vi "HW_Detect_compatible_COM_ports.vi"(0 "Retrieval method (NI-VISA)":enum16{"NI-VISA", "WMIC"}(ring), 1 "Error In":errorcluster) -> (2 "Detected COM ports":T1[](array[typedef]), 3 "Output string from CMD":string="\r\r\n\r\r\n", 4 "Standard error output from CMD":string="No Instance(s) Available.\r\r\n", 5 "Error Out":errorcluster)   [LabVIEW 2018, in "Common_Resources.lvlib"]
uses:
  SubVi's/Controls/CTL_VISA_port_Descr.-Name.ctl
  Common_Resources.lvlib
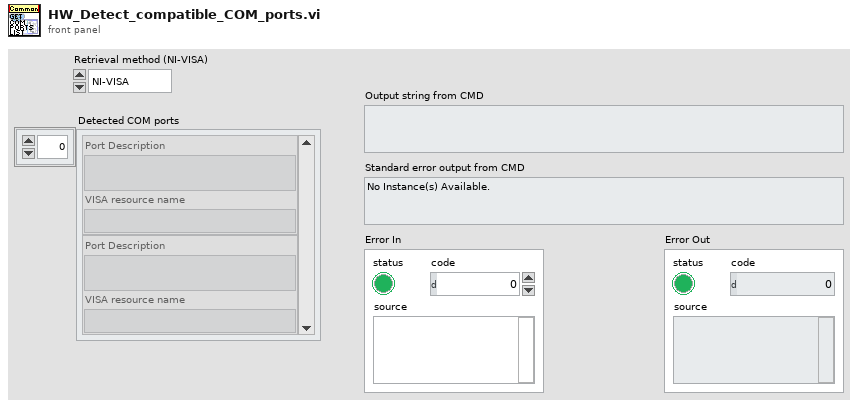
[diagram p1: front panel]
types:
  T1 = typedef "Common_Resources.lvlib/CTL_VISA_port_Descr.-Name.ctl" = cluster{"Port Description":string, "VISA resource name":string}
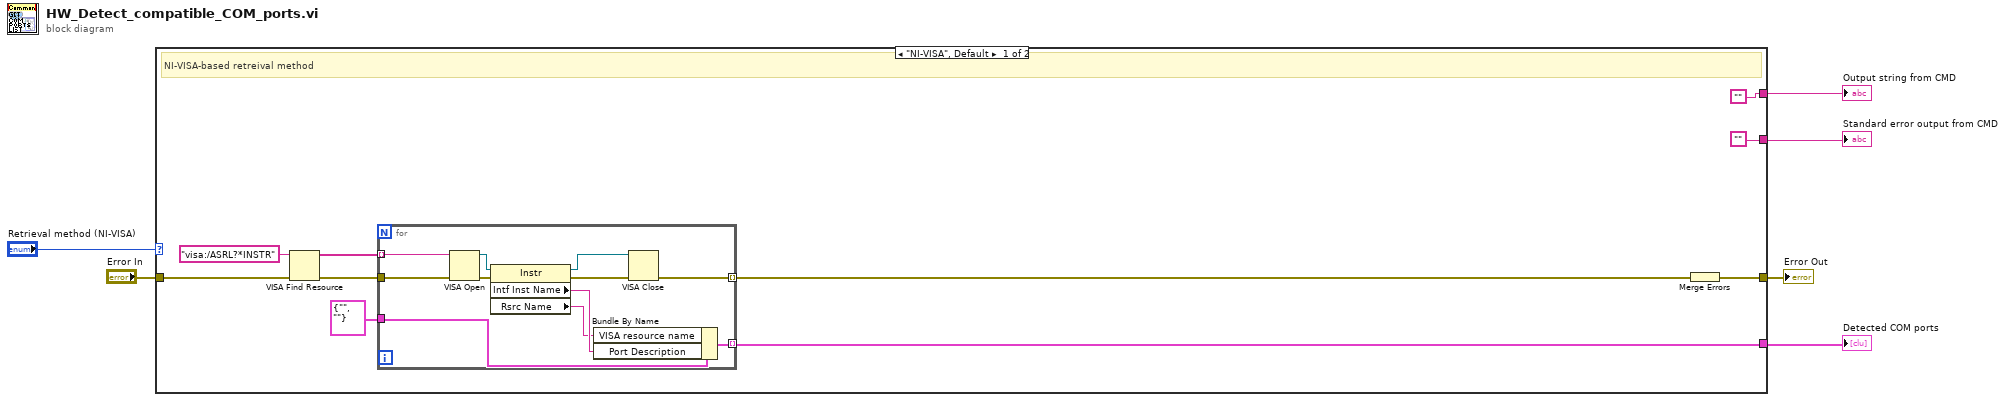
[diagram p0: block diagram]
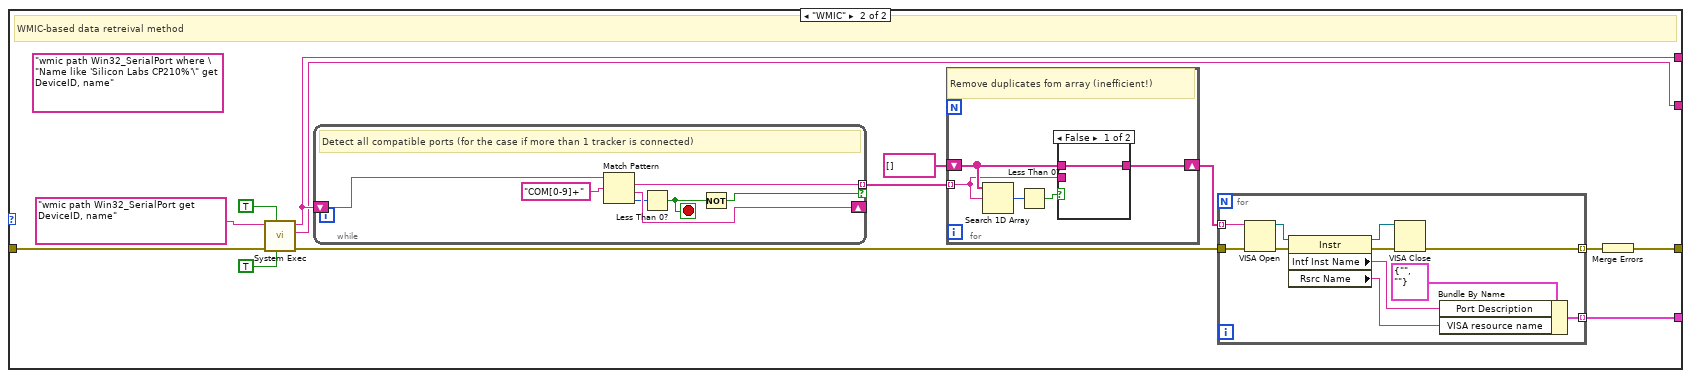
[diagram p2: hidden frame]
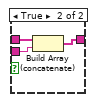
[diagram p3: hidden frame]
diagram:
  n1 = case shown="\"NI-VISA\", Default" "Retrieval method (NI-VISA)" {
    tunnel: "Error In" -> [w14 w37]
    tunnel: [w9 w29] -> w5
    tunnel: ["" w36] -> w4
    tunnel: ["" w35] -> w3
    tunnel: [w8 w28] -> w1
    frame "NI-VISA", Default {
      # "NI-VISA-based retreival method"
      n2 = VISA Find Resource(8:w14, 11:"visa:/ASRL?*INSTR" ("expression (\"?*\")")) -> (0:w12:errorcluster, 3:w15:string[])  [unwired: 1 in, 1 out]
      n3 = for {
        tunnel: w15 -> [w27] mode=indexing
        tunnel: w12 -> [w26]
        tunnel: [w19] -> w8 mode=indexing
        tunnel: [w22] -> w10 mode=indexing
        tunnel: T1 {"Port Description"="", "VISA resource name"=""} ("VISA port  Description-Name pair") -> [w21]
        n4 = VISA Open(error in (no error)=w26, VISA resource name=w27) -> (VISA resource name=w25:refnum<visa-resource-name>, error out=w24:errorcluster)  [unwired: 3 in]
        n5 = property class="Instr"(reference=w25, error in=w24) -> (reference out=w18:refnum<visa-resource-name>, error out=w23:errorcluster, "Intf Inst Name"=w20:string, "Rsrc Name"=w17:string)
        n6 = Bundle By Name(cluster=w21, "VISA resource name"=w17, "Port Description"=w20) -> (w19:T1)
        n7 = VISA Close(VISA resource name=w18, error in (no error)=w23) -> (error out=w22:errorcluster)
      }
      n8 = Merge Errors(w10) -> (w9:errorcluster)
    }
    frame "WMIC" {
      (unwired) "wmic path Win32_SerialPort where \"Name like 'Silicon Labs CP210%'\" get DeviceID, name" ("command line")
      # "WMIC-based data retreival method"
      n9 = call <vilib>:"System Exec.vi"("run minimized? (F)"=TRUE, "wait until completion? (T)"=TRUE, "error in (no error)"=w37, "command line"="wmic path Win32_SerialPort get DeviceID, name") -> ("error out"=w31:errorcluster, "standard error"=w35:string, "standard output"=w36:string)  [unwired: 4 in, 1 out]
      n10 = while {
        shift-right: [w66] -> _
        shift-left: w36 -> [w64]
        tunnel: [w65] -> w34 mode=indexing if=w62
        stop <- w61 stop-if-true
        # "Detect all compatible ports (for the case if more than 1 tracker is connected)"
        n11 = Match Pattern(string=w64, regular expression="COM[0-9]+") -> (match substring=w65:string, after substring=w66:string, offset past match=w63:i32)  [unwired: 1 in, 1 out]
        n12 = Less Than 0?(x=w63) -> (x < 0?=w61:bool)
        n13 = Not(x=w61) -> (.not. x?=w62:bool)
      }
      n14 = for {
        tunnel: w34 -> [w52] mode=indexing
        shift-right: [w53] -> w32
        shift-left: string[] [] -> [w54]
        # "Remove duplicates fom array (inefficient!)"
        n15 = Search 1D Array(1D array=w54, element=w52) -> (index of element=w56:i32)  [unwired: 1 in]
        n16 = Less Than 0?(x=w56) -> (x < 0?=w55:bool)
        n17 = case shown="False" w55 {
          tunnel: w54 -> [w57 w60]
          tunnel: [w57 w59] -> w53
          tunnel: w52 -> [_ w58]
          frame False {
          }
          frame True {
            n18 = Build Array (concatenate)(w60, w58) -> (w59:string[])
          }
        }
      }
      n19 = for {
        tunnel: w32 -> [w51] mode=indexing
        tunnel: w31 -> [w50]
        tunnel: [w44] -> w28 mode=indexing
        tunnel: [w46] -> w30 mode=indexing
        n20 = VISA Open(error in (no error)=w50, VISA resource name=w51) -> (VISA resource name=w49:refnum<visa-resource-name>, error out=w48:errorcluster)  [unwired: 3 in]
        n21 = property class="Instr"(reference=w49, error in=w48) -> (reference out=w43:refnum<visa-resource-name>, error out=w47:errorcluster, "Intf Inst Name"=w42:string, "Rsrc Name"=w41:string)
        n22 = VISA Close(VISA resource name=w43, error in (no error)=w47) -> (error out=w46:errorcluster)
        n23 = Bundle By Name(cluster=T1 {"Port Description"="", "VISA resource name"=""} ("VISA port  Description-Name pair"), "Port Description"=w42, "VISA resource name"=w41) -> (w44:T1)
      }
      n24 = Merge Errors(w30) -> (w29:errorcluster)
    }
  }
  "Error Out" <- w5
  "Output string from CMD" <- w4
  "Standard error output from CMD" <- w3
  "Detected COM ports" <- w1
